vi "Stop Core.vi"(10 "final error code":i32, 11 "DAQ AI in":refnum<class "DAQ AI.lvclass">) -> (3 "DAQ AI out":refnum<class "DAQ AI.lvclass">)   [LabVIEW 2020, in "DAQ AI.lvlib" / "DAQ AI.lvclass"]
doc: "<p>(<strong>Filename</strong>: <span class=\"dnl\">Actor Framework.lvlib:Actor.lvclass:Stop Core.vi</span>)</p>\n<p>Defines what the actor does before it stops. Use the <strong>final error code</strong> input to determine whether the actor shut down in response to an error.</p>\n<p>By default, this method passes the Stop message along to all <a href=\"nihelplauncher://docs/csh?context=lvcore_lvcomm_af_launch_nested_actor\">auto-stop nested actors</a>. A descendant class may override this method to define additional behavior, such as shutting down any processes the actor initiated in its override of the <a href=\"nihelplauncher://docs/csh?context=lvcore_lvcomm_af_actor_core\">Actor Core</a> method.</p>"
uses:
  DAQ AI.lvclass
  DAQ AI.lvclass/DAQ AI.ctl
  <vilib>/ActorFramework/Actor/Actor.lvclass
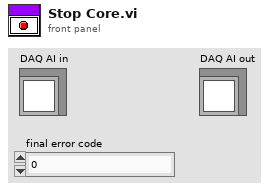
[diagram p1: front panel]
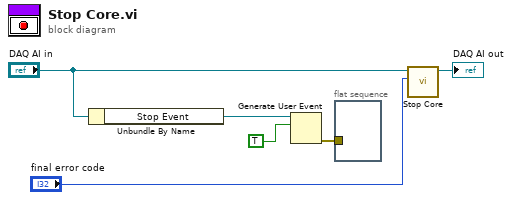
[diagram p0: block diagram]
diagram:
  n1 = Unbundle By Name("DAQ AI in") -> ("Stop Event"=w4:refnum<user-event>)
  n2 = Generate User Event(user event=w4, event data cluster=TRUE ("event data")) -> (error out=w2:errorcluster)  [unwired: 2 in, 1 out]
  n3 = flat-sequence {
    tunnel: w2 -> [_]
    frame #0 {
    }
  }
  n4 = call-parent "Stop Core.vi"("final error code"="final error code", "Actor in"="DAQ AI in") -> ("Actor out"=→"DAQ AI out":refnum<class "DAQ AI.lvclass">)  [unwired: 9 in]
